vi "SECoP-putCommandAnswer_2.vi"(5 "sigma":string, 6 "timestamp":dbl=nan, 7 "command id":u64, 8 "error in (no error)":errorcluster, 9 "value":string, 10 "SECoP error":T1 items=["warn: missing properties"=4, "warn: buffer too small"=3, "warn: custom property"=2, "warn: no description"=1, "success"=0, "error: unknown command"=-1, "error: invalid name"=-2, "error: invalid node"=-3, "error: invalid module"=-4, "error: invalid parameter"=-5, "error: invalid property"=-6, "error: invalid command"=-7, "error: not implemented"=-8, "error: readonly"=-9, "error: no data"=-10, "error: no memory"=-11, "error: not initialized"=-12, "error: invalid value"=-13, "error: missing mandatory prop"=-14, "error: no setter/getter"=-15, "error: no setter"=-16, "error: no getter"=-17, "error: name already in use"=-18], 11 "DLL path (in)":T2) -> (0 "error out":errorcluster, 3 "DLL path (out)":T2)   [LabVIEW 2023, in "SECoP.lvlib"]
doc: "Call <b>\"SECoP-putCommandAnswer_2.vi\"</b>, when \"SECoP-getStoredCommand_2.vi\" or \"SECoP-filterStoredCommand_2.vi\" provided a to do action. You have to provide the read value, value after change or command call result as JSON string. All clients which subscribed to this module should be informed about parameter values.\n\nYour have to call this VI after a successful result from functions before. If your handling was successful, provide a \"success\" error code for this VI. If you encounter an error while handling the action, e.g. communication problem with your device, you should provide a meaningful error code.\n\n<b>DLL path</b> input and output of cluster from \"SECoP-Initialize.vi\"\n<b>command id</b> command id from \"SECoP-getStoredCommand.vi\" or \"SECoP-filterStoredCommand.vi\"\n<b>SECoP error</b> result of the action\n<b>value</b> actual/new value of parameter as JSON string, result of \"do\"-command call (e.g. null for empty replies)\n<b>sigma</b> if applicable, the error bar of the actual/new value of parameter as JSON string (or empty string)\n<b>timestamp</b> time in seconds (with fraction) from 1970/1/1 0:0am of data (or NaN for actual time)"
uses:
  SECoP.lvlib
  SECoP-libraries.ctl
  SECoP-error.ctl
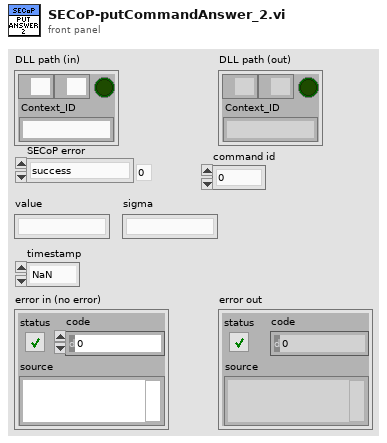
[diagram p1: front panel]
types:
  T1 = typedef "SECoP.lvlib/SECoP-error.ctl" = i32
  T2 = typedef "SECoP.lvlib/SECoP-libraries.ctl" = cluster{"serverDLL":path, "variantDLL":path, "cleanup_mode":bool, "Context_ID":string}
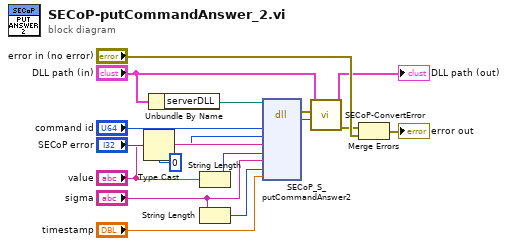
[diagram p0: block diagram]
diagram:
  n1 = Type Cast(type=0 ("SECoP error"), x="SECoP error") -> (*(type *) &x=w2:i32)
  n2 = Unbundle By Name("DLL path (in)") -> ("serverDLL"=w6:path)
  n3 = String Length(string="value") -> (length=w8:i32)
  n4 = String Length(string="sigma") -> (length=w7:i32)
  n5 = dll-call lib="Z:/Praktische Aufgaben/SECoP-LabVIEW2015/32bit/SECoP32.dll" fn="SECoP_S_putCommandAnswer2"(path in=w6, "id"="command id", "SECoP error"=w2, "value"="value", "value size"=w8, "sigma"="sigma", "sigma size"=w7, "timestamp"="timestamp") -> (error out=w5:errorcluster, "return type"=w4:i32)  [unwired: 9 in, 1 out]
  n6 = call "SECoP-ConvertError.vi"("return code"=w4, "error in (no error)"=w5, "DLL path (in)"="DLL path (in)") -> ("error out"=w15:errorcluster, "DLL path (out)"=→"DLL path (out)":T2)  [unwired: 7 in]
  n7 = Merge Errors(w15, "error in (no error)") -> (→"error out":errorcluster)
